vi "Interpolate T to R.vi"(7 "CHANNEL":i32, 8 "TEMPERATURE":dbl, 9 "FILE INFO":T1(array[cluster]), 10 "R/T POINTS":cluster{dbl, dbl}[][](array[cluster]), 11 "CONFIGURATION CLUSTER":T2) -> (1 "RESISTANCE (OHMS)":dbl format="%#_7g", 3 "UNMODIFIED CONFIGURATION CLUSTER":T2, 5 "T PAST CALIBRATION RANGE":bool)   [LabVIEW 2012]
doc: "Calculates resistance from the\ngiven temperature."
panel:
  out "TEMPERATURE UNIT":string
  # "Interpolate T to R.vi"
  # "This VI makes an inverse interpolation from T to R. Its main use will be in temperature control, where it converts the set point, given as temperature, to resistance that can be compared with AVS-47B's output. \n\nThe output of this VI is always in ohms, even if the R/T file lists resistances as log(R).\n\nJust like \"Interpolate R to T.vi\", the R/T points cluster and the file info clusters are needed.\n\nIf the input temperature exceeds the highest or falls below the lowest breakpoint temperature, the error indicator is set true and the limiting breakpoint resistance is returned."
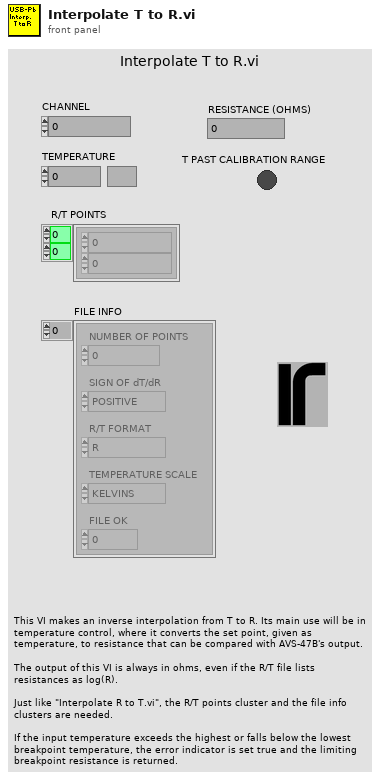
[diagram p1: front panel]
types:
  T1 = cluster{"NUMBER OF POINTS":i32, "SIGN OF dT/dR":enum16{"POSITIVE", "NEGATIVE"}, "R/T FORMAT ":enum16{"R", "LOG(R)"}, "TEMPERATURE SCALE":enum16{"KELVINS", "CELSIUS"}, "FILE OK":i32}[]
  T2 = cluster{"VISA RESOURCE":refnum<visa-resource-name>, "PICOBUS ADDRESS":u8, "DISABLE AL":u8, "REMOTE":u8, "INPUT":u8, "CHANNEL":u8, "RANGE":u8, "EXCITATION":u8, "DISPLAY":u8, "DIGITAL REFERENCE":u16, "SET POINT":dbl, "PROP GAIN":u8, "INTG":u8, "DERIV":u8, "POWER BIAS":u8, "POWER RANGE":u8, "INFO STRING":string, "HEATER RESISTANCE":dbl, "INTERVAL":u8, " SENSOR dR/dT":u8}
  T3 = cluster{"NUMBER OF POINTS":i32, "SIGN OF dT/dR":enum16{"POSITIVE", "NEGATIVE"}, "R/T FORMAT ":enum16{"R", "LOG(R)"}, "TEMPERATURE SCALE":enum16{"KELVINS", "CELSIUS"}, "FILE OK":i32}
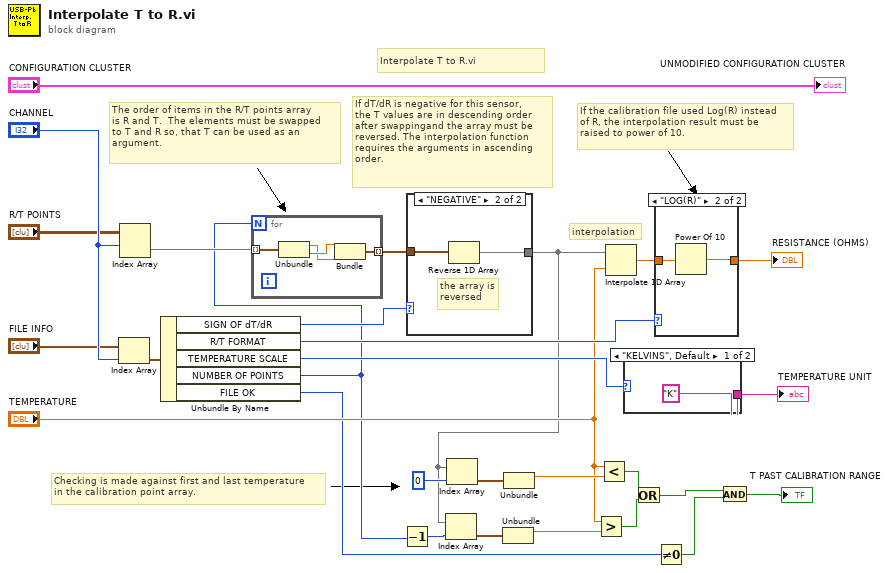
[diagram p0: block diagram]
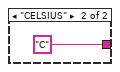
[diagram p2: hidden frame]
diagram:
  # "interpolation"
  # "Checking is made against first and last temperature\nin the calibration point array."
  # "If the calibration file used Log(R) instead\nof R, the interpolation result must be \nraised to power of 10."
  # "If dT/dR is negative for this sensor,\nthe T values are in descending order\nafter swappingand the array must be reversed. The interpolation function requires the arguments in ascending order."
  # "The order of items in the R/T points array\nis R and T.  The elements must be swapped\nto T and R so, that T can be used as an\nargument."
  # "Interpolate T to R.vi"
  n1 = Index Array(array="FILE INFO", index="CHANNEL") -> (element=w23:T3)
  n2 = Index Array(array="R/T POINTS", index (row)="CHANNEL") -> (element=w25:cluster{dbl, dbl}[])  [unwired: 1 in]
  n3 = Unbundle By Name(w23) -> ("SIGN OF dT/dR"=w22:enum16{"POSITIVE", "NEGATIVE"}, "R/T FORMAT"=w21:enum16{"R", "LOG(R)"}, "TEMPERATURE SCALE"=w20:enum16{"KELVINS", "CELSIUS"}, "NUMBER OF POINTS"=w1:i32, "FILE OK"=w4:i32)
  n4 = for {
    N: w1 -> [_]
    tunnel: w25 -> [w32] mode=indexing
    tunnel: [w29] -> w8 mode=indexing
    n5 = Unbundle(w32) -> (w30:dbl, w31:dbl)
    n6 = Bundle(w31, w30) -> (w29:cluster{dbl, dbl})  [unwired: 1 in]
  }
  n7 = Decrement(x=w1) -> (x-1=w17:i32)
  n8 = case shown="\"NEGATIVE\"" w22 {
    tunnel: w8 -> [w33 w35]
    tunnel: [w33 w34] -> w7
    frame "POSITIVE", Default {
    }
    frame "NEGATIVE" {
      # "the array is\nreversed"
      n9 = Reverse 1D Array(array=w35) -> (reversed array=w34:cluster{dbl, dbl}[])
    }
  }
  n10 = Index Array(array=w7, index=w17) -> (element=w15:cluster{dbl, dbl})
  n11 = Index Array(array=w7, index=0) -> (element=w16:cluster{dbl, dbl})
  n12 = Unbundle(w15) -> (w11:dbl)  [unwired: 1 out]
  n13 = Unbundle(w16) -> (w12:dbl)  [unwired: 1 out]
  n14 = Greater?(x="TEMPERATURE", y=w11) -> (0:w13:bool)
  n15 = Less?(x="TEMPERATURE", y=w12) -> (x < y?=w14:bool)
  n16 = Interpolate 1D Array(1:"TEMPERATURE", 2:w7) -> (0:w28:dbl)
  n17 = case shown="\"KELVINS\", Default" w20 {
    tunnel: ["K" "C"] -> w19
    frame "KELVINS", Default {
    }
    frame "CELSIUS" {
    }
  }
  "TEMPERATURE UNIT" <- w19
  n18 = Or(x=w14, y=w13) -> (x .or. y?=w5:bool)
  n19 = case shown="\"LOG(R)\"" w21 {
    tunnel: w28 -> [w38 w40]
    tunnel: [w38 w39] -> w27
    frame "R", Default {
    }
    frame "LOG(R)" {
      n20 = Power Of 10(x=w40) -> (10^x=w39:dbl)
    }
  }
  "RESISTANCE (OHMS)" <- w27
  n21 = Not Equal To 0?(x=w4) -> (x != 0?=w3:bool)
  n22 = And(x=w5, y=w3) -> (x .and. y?=→"T PAST CALIBRATION RANGE":bool)
  "UNMODIFIED CONFIGURATION CLUSTER" <- "CONFIGURATION CLUSTER"
